vi "Configure Position Offset.vi"(8 "error in (no error)":errorcluster, 10 "CCW Position Offset (0.0 rad)":dbl, 11 "Parallax Standard Servo in":refnum<class "Parallax Standard Servo.lvclass">) -> (0 "error out":errorcluster, 3 "Parallax Standard Servo out":refnum<class "Parallax Standard Servo.lvclass">)   [LabVIEW 2019, in "Parallax Standard Servo.lvclass"]
doc: "Configures the counterclockwise software position offset."
uses:
  Parallax Standard Servo.lvclass
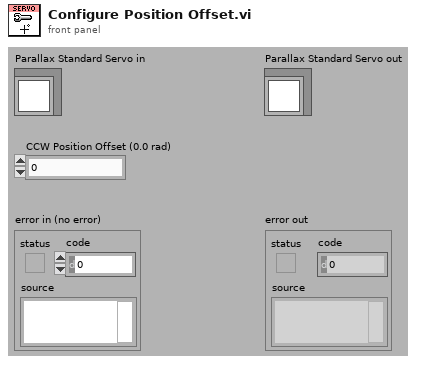
[diagram p1: front panel]
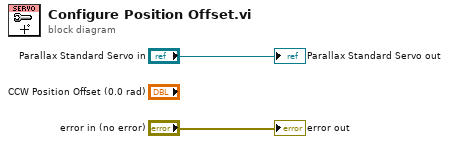
[diagram p0: block diagram]
diagram:
  "error out" <- "error in (no error)"
  "Parallax Standard Servo out" <- "Parallax Standard Servo in"
